vi "Fixed-Point Cast.vi"() -> ()   [LabVIEW 2023]
doc: "This example shows how to use the Fixed-Point to Integer Cast and the Integer to Fixed-Point Cast primitives."
panel:
  out "<+/-, 8, 8>":fxp<+/-,8,8>=-27.0 format="%.0b"
  out "<+, 10, 4>":fxp<+,10,4>=15.578125 format="%.0b"
  in  "<+/-, 6, 3>":fxp<+/-,6,3>=-4.0 format="%.0b"
  out "I8":i8=-19 format="%.0b"
  in  "<+, 8, 8>":fxp<+,8,8>=45.0 format="%.0b"
  out "U8":u8=45 format="%.0b"
  out "<+/-, 6, 6>":fxp<+/-,6,6>=-28.0 format="%.0b"
  in  "I8 2":i8=-27 format="%.0b"
  in  "Stop":bool
  # "Overview: Demonstrates how the Fixed-Point to Integer Cast and Integer to Fixed-Point Cast functions operate.\nInstructions:\n1. Run the VI.\n2. Examine the different cases.\n3. Click Stop to stop the VI."
  # "This case shows an integer being cast to a fixed-point type with the default configuration, with a wired in configuration and with a manually configured output."
  # "This case shows how integer output type is calculated so that it will be the smallest type that will hold all of the input bits."
  # "The bits are copied over exactly and the data is interpreted as the new type."
  # "The bits are copied over exactly and the data is interpreted as the new type."
  # "Default Configuration"
  # "Property Page Configuration"
  # "Since the fixed-point number is represented using two's complement, the most significant digits of the output will be sign extended"
  # "Wired Configuration"
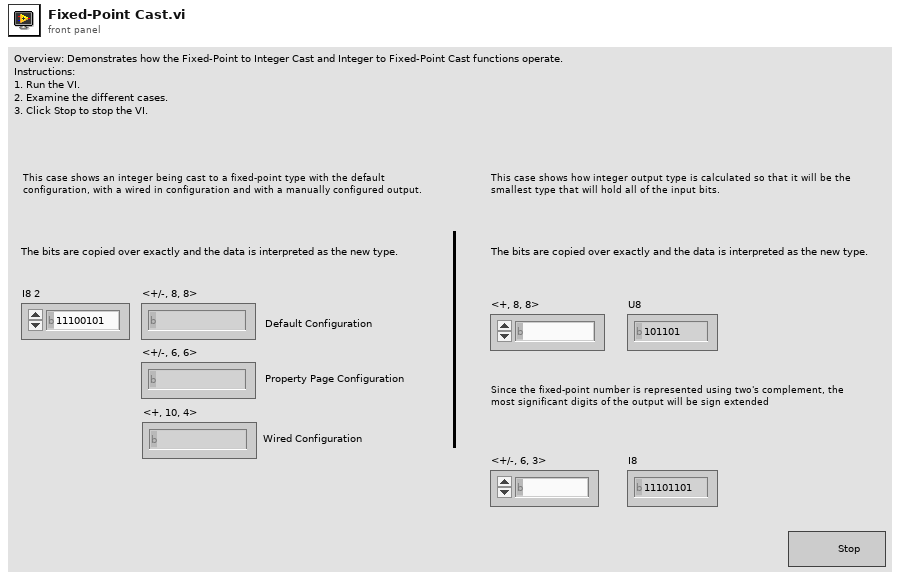
[diagram p1: front panel]
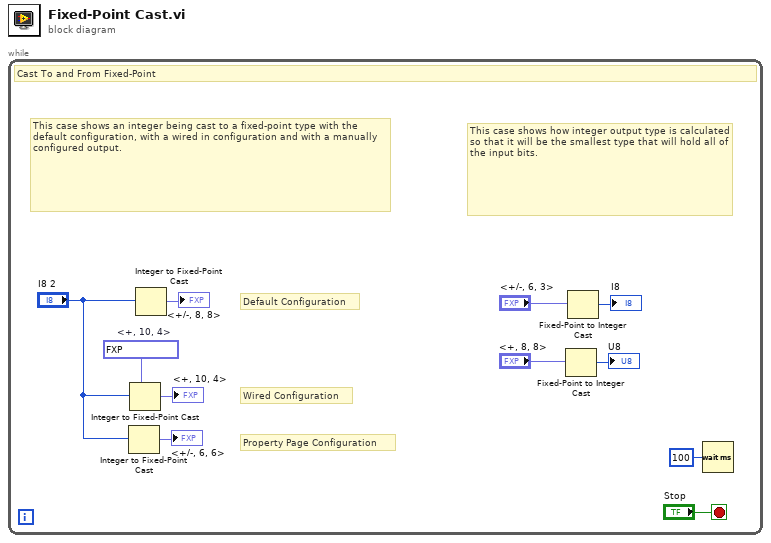
[diagram p0: block diagram]
diagram:
  n1 = while {
    stop <- "Stop" stop-if-true
    w5 = fxp<+,10,4> 0.0  # <+, 10, 4>
    # "This case shows an integer being cast to a fixed-point type with the default configuration, with a wired in configuration and with a manually configured output."
    # "Property Page Configuration"
    # "Wired Configuration"
    # "Default Configuration"
    # "This case shows how integer output type is calculated so that it will be the smallest type that will hold all of the input bits."
    # "Cast To and From Fixed-Point"
    n2 = Integer to Fixed-Point Cast(integer="I8 2") -> (fixed-point=→"<+/-, 6, 6>":fxp<+/-,6,6>)  [unwired: 1 in]
    n3 = Integer to Fixed-Point Cast(fixed-point type=w5, integer="I8 2") -> (fixed-point=→"<+, 10, 4>":fxp<+,10,4>)
    n4 = Integer to Fixed-Point Cast(integer="I8 2") -> (fixed-point=→"<+/-, 8, 8>":fxp<+/-,8,8>)  [unwired: 1 in]
    n5 = Fixed-Point to Integer Cast(1:"<+, 8, 8>") -> (0:→"U8":u8)
    n6 = Fixed-Point to Integer Cast(1:"<+/-, 6, 3>") -> (0:→"I8":i8)
    n7 = Wait (ms)(milliseconds to wait=u32 100 ("millisecond multiple")) -> ()  [unwired: 1 out]
  }
